vi "实验5_1.vi"() -> ()   [LabVIEW 2018]
panel:
  out "日期":string
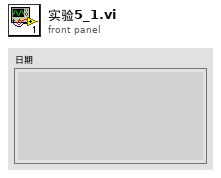
[diagram p1: front panel]
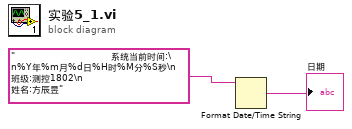
[diagram p0: block diagram]
diagram:
  n1 = Format Date/Time String(time format string (%c)="                                系统当前时间:\n%Y年%m月%d日%H时%M分%S秒\n                              班级:测控1802\n                              姓名:方辰昱") -> (date/time string=→"日期":string)  [unwired: 2 in]
